vi "subPlotSpectrum.vi"(0 "Spectrum to Plot":cluster{"f0":dbl, "df":dbl, "IQ":dbl[]}, 7 "Frame Parameters":T1={"IQ Rate"=0.0, "Frames"=0, "Length of Subset"=0, "Start Index of Subset"=0, "Start Carrier [Hz]"=88500000.0, "Stop Carrier [Hz]"=107700000.0, "Acq Duration [sec]"=0.01} {"Acq Duration [sec]" min=0.0 step=0.001 format="%#.6p"; "Stop Carrier [Hz]" min=50000000.0 max=6000000000.0 step=1000.0 format="%#.15p"; "Start Carrier [Hz]" min=50000000.0 max=6000000000.0 step=1000.0 format="%#.15p"}, 9 "window properties":cluster{"eq noise BW":dbl, "coherent gain":dbl}, 12 "Display":T2) -> (4 "Spectrum to Plot":cluster{"f0":dbl, "df":dbl, "IQ":dbl[]})   [LabVIEW 2015]
uses:
  subFrameParams.ctl
  <vilib>/Analysis/NI_AALPro.lvlib
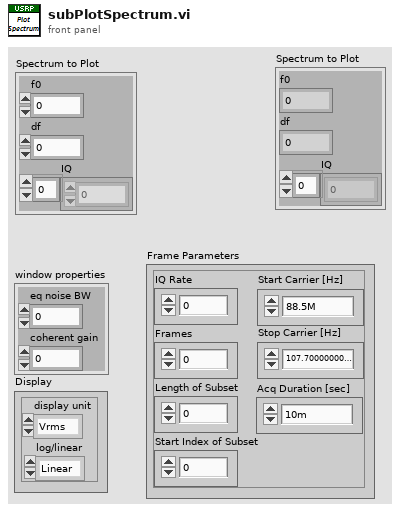
[diagram p1: front panel]
types:
  T1 = typedef "subFrameParams.ctl" = cluster{"IQ Rate":dbl, "Frames":i32, "Length of Subset":i32, "Start Index of Subset":i32, "Start Carrier [Hz]":dbl, "Stop Carrier [Hz]":dbl, "Acq Duration [sec]":dbl}
  T2 = cluster{"display unit":enum32{"Vrms", "Vpk", "Vrms^2", "Vpk^2", "Vrms/rtHz", "Vpk/rtHz", "Vrms^2/Hz", "Vpk^2/Hz"}, "log/linear":enum16{"Linear", "dB", "dBm"}}
  T3 = enum16{"Power (Vrms^2)", "Amplitude (Vrms)", "Gain (amplitude ratio)"}
  T4 = enum32{"Vrms", "Vpk", "Vrms^2", "Vpk^2", "Vrms/rtHz", "Vpk/rtHz", "Vrms^2/Hz", "Vpk^2/Hz"}
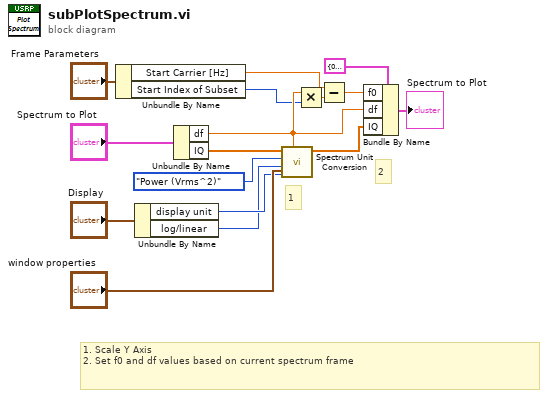
[diagram p0: block diagram]
diagram:
  # "2"
  # "1"
  # "1. Scale Y Axis\n2. Set f0 and df values based on current spectrum frame"
  n1 = Unbundle By Name("Frame Parameters") -> ("Start Carrier [Hz]"=w2:dbl, "Start Index of Subset"=w3:i32)
  n2 = Unbundle By Name("Display") -> ("display unit"=w9:T4, "log/linear"=w8:enum16{"Linear", "dB", "dBm"})
  n3 = Unbundle By Name("Spectrum to Plot") -> ("df"=w7:dbl, "IQ"=w5:dbl[])
  n4 = call <vilib>:"Spectrum Unit Conversion.vi"("window constants"="window properties", "df"=w7, "display unit"=w9, "log/linear"=w8, "spectrum type"=T3."Power (Vrms^2)", "Spectrum in"=w5) -> ("Spectrum out"=w13:dbl[])  [unwired: 4 in, 1 out]
  n5 = Multiply(x=w7, y=w3) -> (x*y=w16:dbl)
  n6 = Subtract(x=w2, y=w16) -> (x-y=w15:dbl)
  n7 = Bundle By Name(cluster=cluster{"f0":dbl, "df":dbl, "IQ":dbl[]} {"f0"=0.0, "df"=0.0, "IQ"=[]} ("real part"), "f0"=w15, "df"=w7, "IQ"=w13) -> (→"Spectrum to Plot":cluster{"f0":dbl, "df":dbl, "IQ":dbl[]})
